vi "Get Transceivers.vi"(11 "Framework in":refnum<class "Framework.lvclass">) -> (2 "Transceivers":refnum<class "Transceiver.lvclass">[](array[class]), 3 "Framework out":refnum<class "Framework.lvclass">)   [LabVIEW 2017, in "DSF Core.lvlib" / "Framework.lvclass"]
uses:
  Framework.lvclass
  Transceiver/Transceiver.lvclass
  Framework.lvclass/Framework.ctl
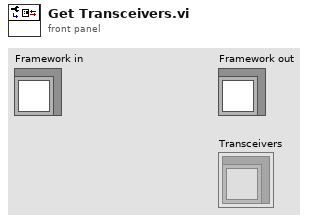
[diagram p1: front panel]
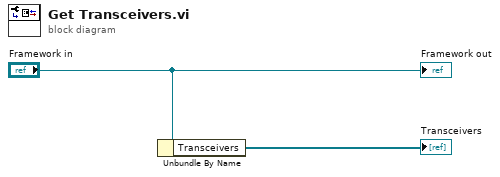
[diagram p0: block diagram]
diagram:
  n1 = Unbundle By Name("Framework in") -> ("Transceivers"=→"Transceivers":refnum<class "Transceiver.lvclass">[])
  "Framework out" <- "Framework in"
